vi "Notifier Obtain.vi"(8 "error in (no error)":errorcluster, 10 "Notifier Name":string, 11 "Messaging in":refnum<class "Messaging.lvclass">) -> (0 "error out":errorcluster, 3 "Messaging out":refnum<class "Messaging.lvclass">)   [LabVIEW 2023, in "Messaging.lvclass"]
uses:
  Messaging.lvclass
  Msg.Data.ctl
  Messaging.lvclass/Messaging.ctl
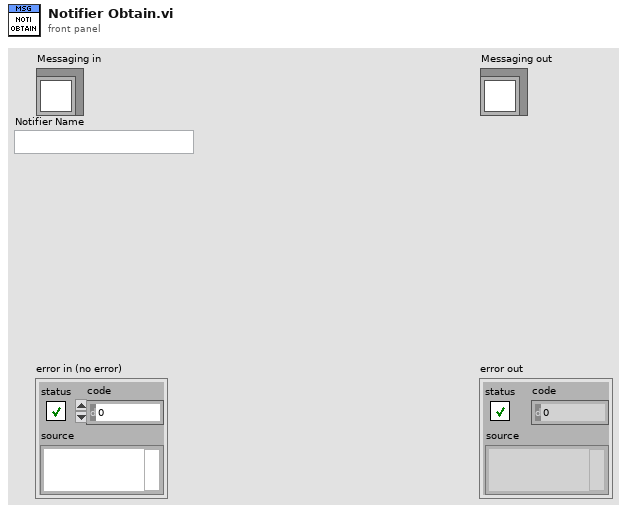
[diagram p1: front panel]
types:
  T1 = typedef "Messaging.lvclass/Msg.Data.ctl" = cluster{"Message":string, "Data":variant}
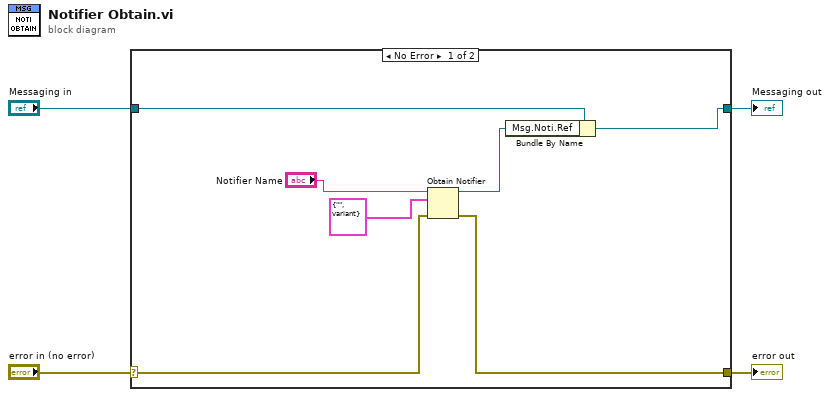
[diagram p0: block diagram]
diagram:
  n1 = case shown="No Error" "error in (no error)" {
    selector: "error in (no error)" -> [w9 w13]
    tunnel: [w6 w13] -> w3
    tunnel: [w5 w12] -> w1
    tunnel: "Messaging in" -> [w8 w12]
    frame No Error {
      n2 = Obtain Notifier(name (unnamed)="Notifier Name", notification data type=T1 {"Message"="", "Data"=variant} ("Msg.Q.Data"), error in (no error)=w9) -> (notifier out=w7:refnum<notifier>, error out=w6:errorcluster)  [unwired: 1 in, 1 out]
      n3 = Bundle By Name(cluster=w8, "Msg.Noti.Ref"=w7) -> (w5:refnum<class "Messaging.lvclass">)
    }
    frame Error {
    }
  }
  "error out" <- w3
  "Messaging out" <- w1
